vi "ROI entry-Offset limits.vi"(9 "Offsets cluster in in":cluster{"X offset":dbl, "Y offset":dbl}, 10 "Function":T1=enum."Offset all ROI", 11 "ROI setup in":T2[](array[typedef]) {"Apparent Frame Size" format="%#_6f"; "Original FOV (um)" format="%#_6f"; "Pixels per miniscan" format="%#_6f"; "Dwell Time per pixel" format="%#_6f"; "Resolution" format="%#_6f"; "ROI group ID" format="%#_6f"; "Laser Power (%)" format="%#_6f"; "Zoom" format="%#_6f"; "Frame Size" format="%#_6f"; "Number of lines" format="%#_6f"; "Composite ID" format="%#_6f"; "Angle (deg)" format="%#_6f"; "ROI Time (ns)" format="%#_6f"; "ROI ID" format="%#_6f"; "Pixels in ROI" format="%#_6f"; "ROI index" format="%#_6f"; "Z stop" format="%#_6f"; "Y stop" format="%#_6f"; "X stop" format="%#_6f"; "Z start" format="%#_6f"; "X start" format="%#_6f"; "Y start" format="%#_6f"}) -> (3 "Offsets cluster out":T3)   [LabVIEW 2020]
uses:
  Typedefs/Offset adjustments cluster.ctl
  Visualisation/Functional Imaging Viewer/Typedefs/ROI parameters data type.ctl
  Typedefs/ROI management FG states.ctl
  <userlib>/_OpenG.lib/array/array.llb/Conditional Auto-Indexing Tunnel (DBL)__ogtk.vi
panel:
  out "Y Stop > Max":bool[](array[boolean])
  out "Y Start <0":bool[](array[boolean])
  out "X Stop > Max":bool[](array[boolean])
  out "X Start <0":bool[](array[boolean])
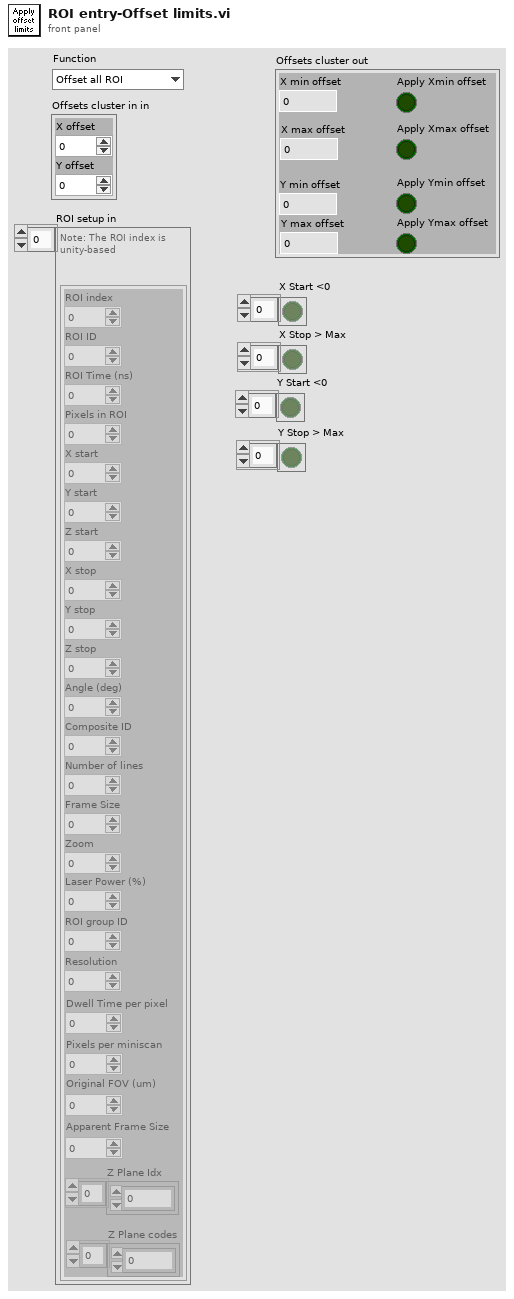
[diagram p1: front panel]
types:
  T1 = typedef "ROI management FG states.ctl" = enum16{"Read", "Write", "Write-from dataset", "Clear Last", "Clear All", "Delete ROI", "Update ROIs time", "Reload last ROI set", "Modify ROI Parameters", "Offset all ROI", "Offset visible ROI", "Modify Dwell Time", "Modify Laser Power"}
  T2 = typedef "ROI parameters data type.ctl" = cluster{"ROI index":dbl, "ROI ID":dbl, "ROI Time (ns)":dbl, "Pixels in ROI":dbl, "X start":dbl, "Y start":dbl, "Z start":dbl, "X stop":dbl, "Y stop":dbl, "Z stop":dbl, "Angle (deg)":dbl, "Composite ID":dbl, "Number of lines":dbl, "Frame Size":dbl, "Zoom":dbl, "Laser Power (%)":dbl, "ROI group ID":dbl, "Resolution":dbl, "Dwell Time per pixel":dbl, "Pixels per miniscan":dbl, "Original FOV (um)":dbl, "Apparent Frame Size":dbl, "Z Plane Idx":i32[], "Z Plane codes":i32[]}
  T3 = typedef "Offset adjustments cluster.ctl" = cluster{"X min offset":dbl, "Apply Xmin offset":bool, "X max offset":dbl, "Apply Xmax offset":bool, "Y min offset":dbl, "Apply Ymin offset":bool, "Y max offset":dbl, "Apply Ymax offset":bool}
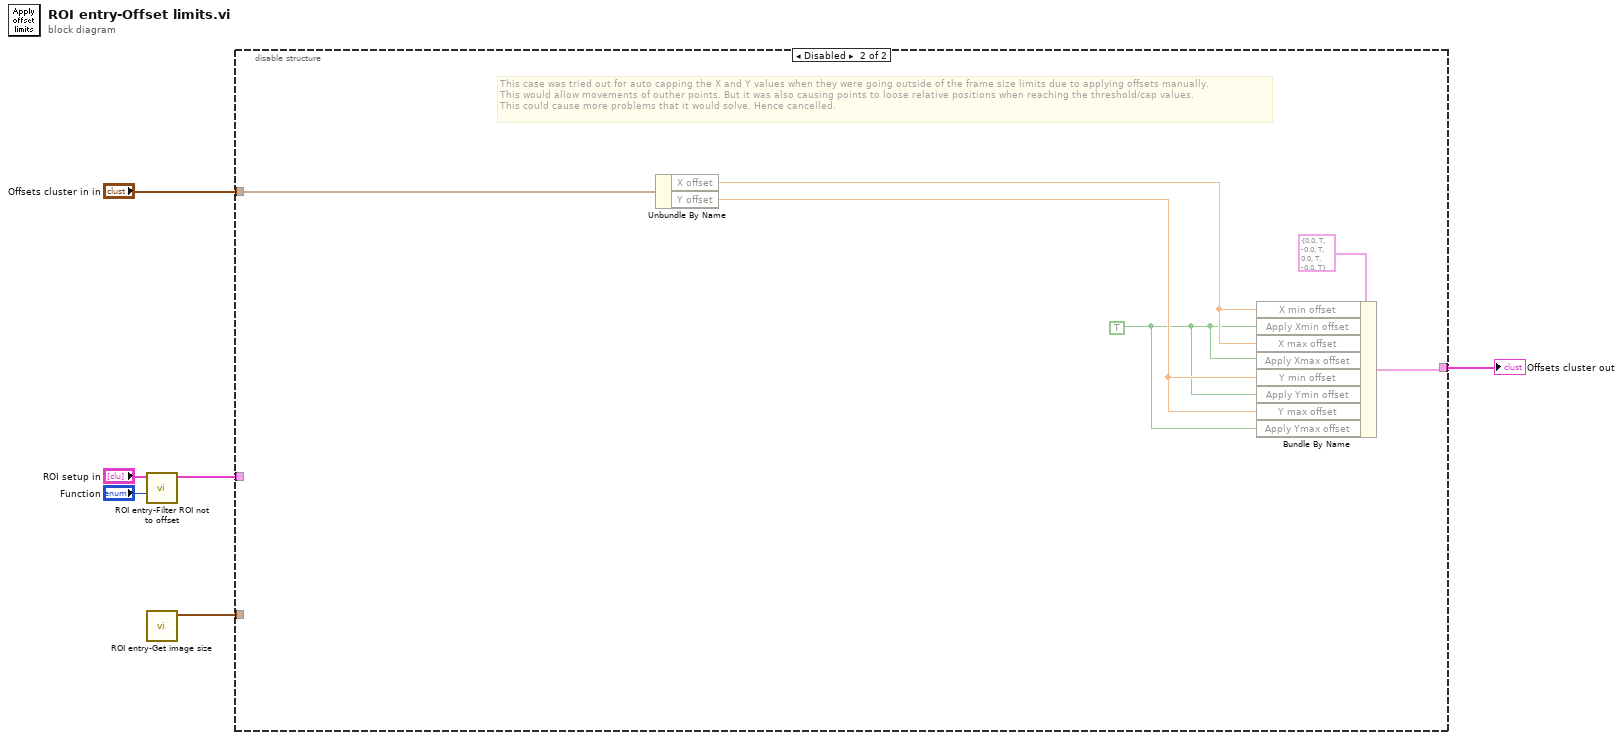
[diagram p0: block diagram]
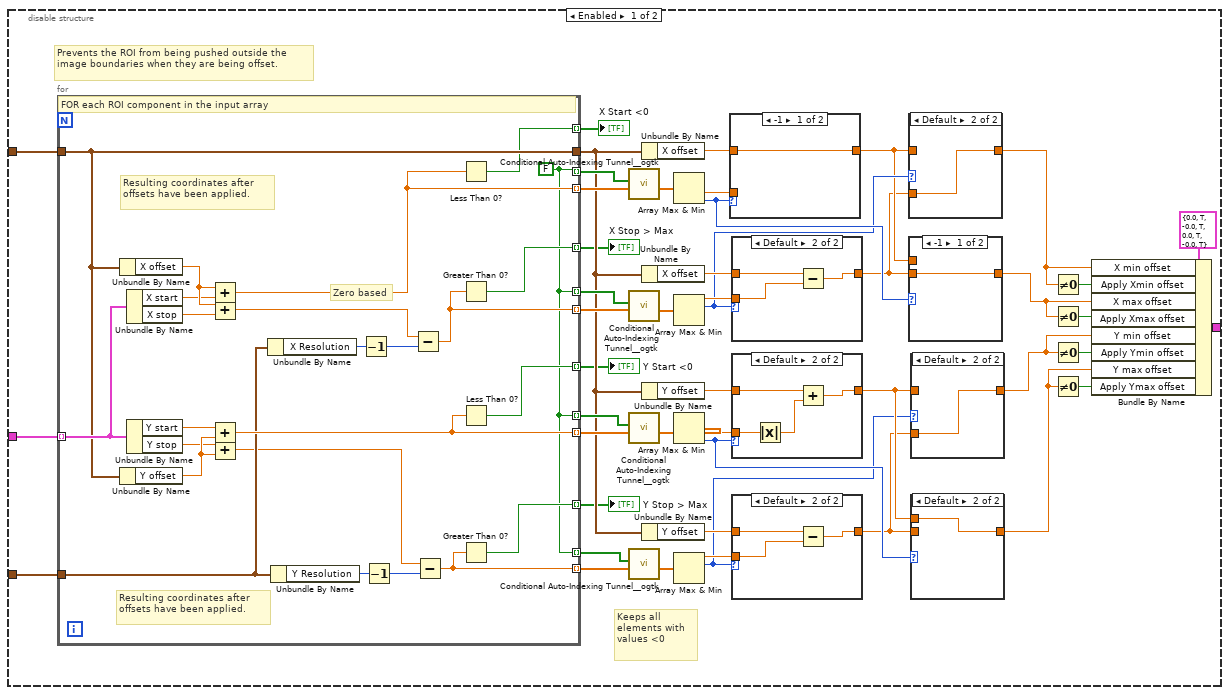
[diagram p2: hidden frame]
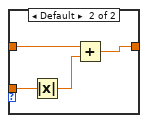
[diagram p10: hidden frame]
diagram:
  n1 = call "ROI entry-Filter ROI not to offset.vi"("Function"="Function", "ROI setup in"="ROI setup in") -> ("Filtered ROI"=w2:T2[])  [unwired: 9 in]
  n2 = call "ROI entry-Get image size.vi"() -> ("Image size"=w5:cluster{"X Resolution":i32, "Y Resolution":i32})  [unwired: 10 in, 1 out]
  n3 = disable-structure shown="Disabled" {
    disable-tunnel: "Offsets cluster in in" -> [w52 w106]
    disable-tunnel: w5 -> [w51 _]
    disable-tunnel: [w42 w107] -> w4
    disable-tunnel: w2 -> [w11 _]
    frame Enabled {
      # "Keeps all elements with values <0"
      # "Prevents the ROI from being pushed outside the image boundaries when they are being offset."
      n4 = for {
        tunnel: w52 -> [w88]
        tunnel: w11 -> [w93] mode=indexing
        tunnel: [w88] -> w29
        tunnel: [w92] -> w45 mode=indexing
        tunnel: [w89] -> w46 mode=indexing
        tunnel: [w96] -> w48 mode=indexing
        tunnel: [w97] -> w50 mode=indexing
        tunnel: w51 -> [w90]
        tunnel: [w79] -> w49 mode=indexing
        tunnel: [w79] -> w47 mode=indexing
        tunnel: [w79] -> w44 mode=indexing
        tunnel: [w79] -> w43 mode=indexing
        tunnel: [w83] -> w10 mode=indexing
        tunnel: [w82] -> w9 mode=indexing
        tunnel: [w81] -> w8 mode=indexing
        tunnel: [w80] -> w7 mode=indexing
        w79 = FALSE
        # "Resulting coordinates after offsets have been applied."
        # "Resulting coordinates after offsets have been applied."
        # "Zero based"
        # "FOR each ROI component in the input array"
        n5 = Unbundle By Name(w88) -> ("X offset"=w102:dbl)
        n6 = Unbundle By Name(w88) -> ("Y offset"=w101:dbl)
        n7 = Unbundle By Name(w93) -> ("X start"=w95:dbl, "X stop"=w94:dbl)
        n8 = Unbundle By Name(w93) -> ("Y start"=w100:dbl, "Y stop"=w99:dbl)
        n9 = Add(x=w102, y=w95) -> (x+y=w92:dbl)
        n10 = Add(x=w102, y=w94) -> (x+y=w84:dbl)
        n11 = Add(x=w100, y=w101) -> (x+y=w96:dbl)
        n12 = Add(x=w99, y=w101) -> (x+y=w87:dbl)
        n13 = Unbundle By Name(w90) -> ("X Resolution"=w91:i32)
        n14 = Unbundle By Name(w90) -> ("Y Resolution"=w98:i32)
        n15 = Decrement(x=w91) -> (x-1=w85:i32)
        n16 = Decrement(x=w98) -> (x-1=w86:i32)
        n17 = Subtract(x=w84, y=w85) -> (x-y=w89:dbl)
        n18 = Subtract(x=w87, y=w86) -> (x-y=w97:dbl)
        n19 = Less Than 0?(x=w92) -> (x < 0?=w83:bool)
        n20 = Greater Than 0?(x=w89) -> (x > 0?=w82:bool)
        n21 = Less Than 0?(x=w96) -> (x < 0?=w81:bool)
        n22 = Greater Than 0?(x=w97) -> (x > 0?=w80:bool)
      }
      "X Start <0" <- w10
      "X Stop > Max" <- w9
      "Y Start <0" <- w8
      "Y Stop > Max" <- w7
      n23 = call-poly <userlib>:"Conditional Auto-Indexing Tunnel__ogtk.vi"("Array in"=w45, "Elements to keep"=w44) -> ("Filtered Array out"=w41:dbl[])  [unwired: 5 in]
      n24 = call-poly <userlib>:"Conditional Auto-Indexing Tunnel__ogtk.vi"("Array in"=w46, "Elements to keep"=w43) -> ("Filtered Array out"=w38:dbl[])  [unwired: 5 in]
      n25 = call-poly <userlib>:"Conditional Auto-Indexing Tunnel__ogtk.vi"("Array in"=w48, "Elements to keep"=w47) -> ("Filtered Array out"=w39:dbl[])  [unwired: 5 in]
      n26 = call-poly <userlib>:"Conditional Auto-Indexing Tunnel__ogtk.vi"("Array in"=w50, "Elements to keep"=w49) -> ("Filtered Array out"=w37:dbl[])  [unwired: 5 in]
      n27 = Unbundle By Name(w29) -> ("X offset"=w32:dbl)
      n28 = Unbundle By Name(w29) -> ("X offset"=w28:dbl)
      n29 = Unbundle By Name(w29) -> ("Y offset"=w31:dbl)
      n30 = Unbundle By Name(w29) -> ("Y offset"=w26:dbl)
      n31 = Array Max & Min(array=w41) -> (min value=w40:dbl, min index (indices)=w24:i32)  [unwired: 2 out]
      n32 = Array Max & Min(array=w38) -> (max value=w27:dbl, max index (indices)=w22:i32)  [unwired: 2 out]
      n33 = Array Max & Min(array=w39) -> (min value=w30:dbl, min index (indices)=w17:i32)  [unwired: 2 out]
      n34 = Array Max & Min(array=w37) -> (max value=w25:dbl, max index (indices)=w15:i32)  [unwired: 2 out]
      n35 = case shown="-1" w24 {
        tunnel: w40 -> [_ w78]
        tunnel: [w74 w75] -> w21
        tunnel: w32 -> [w74 w76]
        frame -1 {
        }
        frame Default {
          n36 = Absolute Value(x=w78) -> (abs(x)=w77:dbl)
          n37 = Add(x=w76, y=w77) -> (x+y=w75:dbl)
        }
      }
      n38 = case shown="Default" w22 {
        tunnel: [w65 w67] -> w20
        tunnel: w28 -> [w65 w68]
        tunnel: w27 -> [_ w66]
        frame -1 {
        }
        frame Default {
          n39 = Subtract(x=w68, y=w66) -> (x-y=w67:dbl)
        }
      }
      n40 = case shown="Default" w17 {
        tunnel: w30 -> [_ w73]
        tunnel: [w69 w70] -> w16
        tunnel: w31 -> [w69 w71]
        frame -1 {
        }
        frame Default {
          n41 = Absolute Value(x=w73) -> (abs(x)=w72:dbl)
          n42 = Add(x=w71, y=w72) -> (x+y=w70:dbl)
        }
      }
      n43 = case shown="Default" w15 {
        tunnel: [w61 w63] -> w14
        tunnel: w26 -> [w61 w64]
        tunnel: w25 -> [_ w62]
        frame -1 {
        }
        frame Default {
          n44 = Subtract(x=w64, y=w62) -> (x-y=w63:dbl)
        }
      }
      n45 = case shown="Default" w22 {
        tunnel: w21 -> [w57 _]
        tunnel: [w57 w58] -> w13
        tunnel: w20 -> [_ w58]
        frame -1 {
        }
        frame Default {
        }
      }
      n46 = case shown="-1" w24 {
        tunnel: w20 -> [w59 _]
        tunnel: [w59 w60] -> w23
        tunnel: w21 -> [_ w60]
        frame -1 {
        }
        frame Default {
        }
      }
      n47 = case shown="Default" w15 {
        tunnel: w16 -> [w53 _]
        tunnel: [w53 w54] -> w19
        tunnel: w14 -> [_ w54]
        frame -1 {
        }
        frame Default {
        }
      }
      n48 = case shown="Default" w17 {
        tunnel: w14 -> [w55 _]
        tunnel: [w55 w56] -> w18
        tunnel: w16 -> [_ w56]
        frame -1 {
        }
        frame Default {
        }
      }
      n49 = Not Equal To 0?(x=w13) -> (x != 0?=w36:bool)
      n50 = Not Equal To 0?(x=w23) -> (x != 0?=w35:bool)
      n51 = Not Equal To 0?(x=w19) -> (x != 0?=w33:bool)
      n52 = Not Equal To 0?(x=w18) -> (x != 0?=w34:bool)
      n53 = Bundle By Name(cluster=T3 {"X min offset"=0.0, "Apply Xmin offset"=TRUE, "X max offset"=-0.0, "Apply Xmax offset"=TRUE, "Y min offset"=0.0, "Apply Ymin offset"=TRUE, "Y max offset"=-0.0, "Apply Ymax offset"=TRUE} ("Offsets cluster out"), "X min offset"=w13, "Apply Xmin offset"=w36, "X max offset"=w23, "Apply Xmax offset"=w35, "Y min offset"=w19, "Apply Ymin offset"=w33, "Y max offset"=w18, "Apply Ymax offset"=w34) -> (w42:T3)
    }
    frame Disabled {
      w103 = TRUE
      # "This case was tried out for auto capping the X and Y values when they were going outside of the frame size limits due to applying offsets manually.\nThis would allow movements of outher points. But it was also causing points to loose relative positions when reaching the threshold/cap values. \nThis could cause more problems that it would solve. Hence cancelled."
      n54 = Unbundle By Name(w106) -> ("X offset"=w105:dbl, "Y offset"=w104:dbl)
      n55 = Bundle By Name(cluster=T3 {"X min offset"=0.0, "Apply Xmin offset"=TRUE, "X max offset"=-0.0, "Apply Xmax offset"=TRUE, "Y min offset"=0.0, "Apply Ymin offset"=TRUE, "Y max offset"=-0.0, "Apply Ymax offset"=TRUE} ("Offsets cluster out"), "X min offset"=w105, "Apply Xmin offset"=w103, "X max offset"=w105, "Apply Xmax offset"=w103, "Y min offset"=w104, "Apply Ymin offset"=w103, "Y max offset"=w104, "Apply Ymax offset"=w103) -> (w107:T3)
    }
  }
  "Offsets cluster out" <- w4
